vi "FTW-Collection-KeyValue-JSON-Deserialize.vi"(0 "Serialized Key-Value Pair":string, 11 "error in":errorcluster) -> (4 "Key-Value Pair":T1, 6 "Valid Structure":bool, 15 "error out":errorcluster)   [LabVIEW 2014]
uses:
  FTW-Collection-KeyValuePair.ctl
  Regex/FTW-Regex.vi
  JSON/FTW-JSON-RegexHeader.vi
  Error/FTW-ERR-ThrowError.vi
panel:
  # "Inputs"
  # "Outputs"
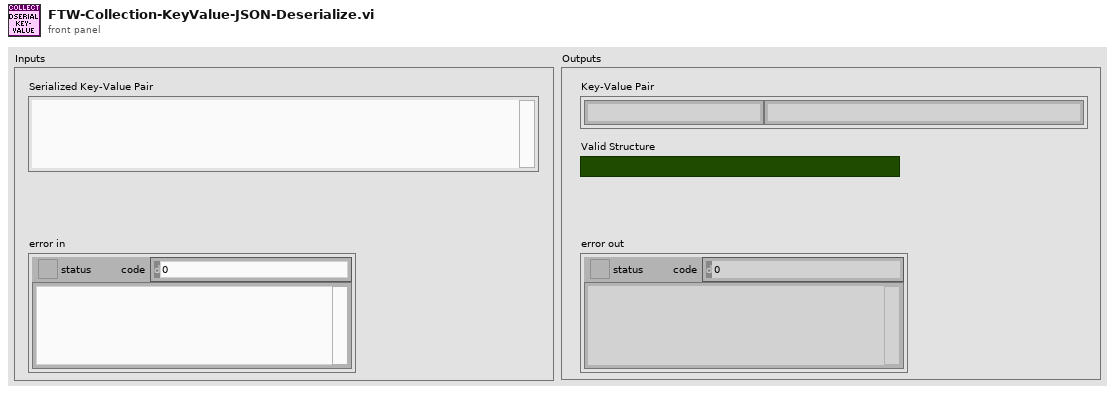
[diagram p1: front panel]
types:
  T1 = typedef "FTW-Collection-KeyValuePair.ctl" = cluster{"Key":string, "Value":string}
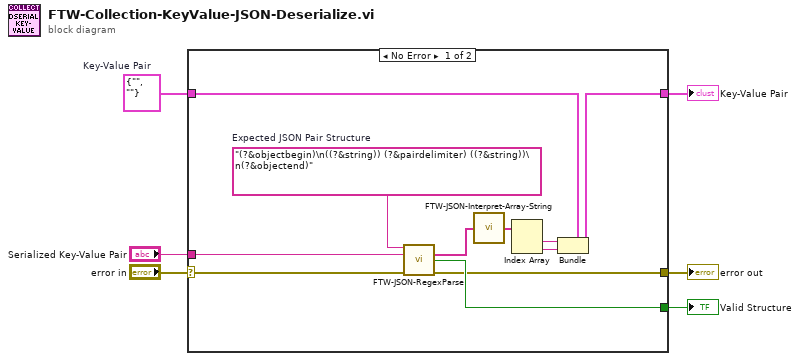
[diagram p0: block diagram]
diagram:
  w4 = T1 {"Key"="", "Value"=""}  # Key-Value Pair
  n1 = case shown="No Error" "error in" {
    selector: "error in" -> [w11 w18]
    tunnel: [w17 w19] -> w5
    tunnel: w4 -> [w16 w19]
    tunnel: [w12 w18] -> w3
    tunnel: "Serialized Key-Value Pair" -> [w14 _]
    tunnel: [w13 _] -> w1
    frame No Error {
      w15 = "(?&objectbegin)\n((?&string)) (?&pairdelimiter) ((?&string))\n(?&objectend)"  # Expected JSON Pair Structure
      n2 = call "FTW-JSON-RegexParse.vi"("Regular Expression using JSON subroutines"=w15, "Input String"=w14, "error in"=w11) -> ("Submatches"=w10:string[], "Found Match?"=w13:bool, "error out"=w12:errorcluster)  [unwired: 8 in, 2 out]
      n3 = call "FTW-JSON-Interpret-Array-String.vi"("Escaped JSON Strings"=w10) -> ("LabVIEW Strings"=w9:string[])
      n4 = Index Array(array=w9) -> (element #1=w8:string, element #2=w7:string)  [unwired: 2 in]
      n5 = Bundle(cluster=w16, "Key"=w8, "Value"=w7) -> (w17:T1)
    }
    frame Error {
    }
  }
  "Key-Value Pair" <- w5
  "error out" <- w3
  "Valid Structure" <- w1
